vi "Compre String without Case Sensitive .vi"(10 "String B":string, 11 "String A":string) -> (3 "A=B?":bool)   [LabVIEW 2021, in "CANOpen Addon System Explorer.lvlib"]
uses:
  CANOpen Addon System Explorer.lvlib
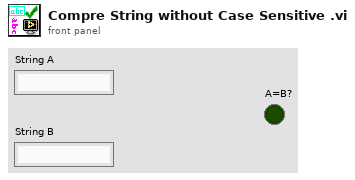
[diagram p1: front panel]
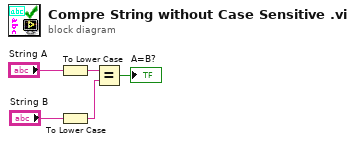
[diagram p0: block diagram]
diagram:
  n1 = To Lower Case(string="String A") -> (all lower case string=w3:string)
  n2 = To Lower Case(string="String B") -> (all lower case string=w2:string)
  n3 = Equal?(x=w3, y=w2) -> (x = y?=→"A=B?":bool)
